vi "Hahn 2 Pulse Sequence Generator.vi"(4 "MW Delay":dbl, 5 "Optical Pulse Sequence":T1(array[cluster]), 6 "Tau' step size 2":dbl, 7 "No. Instructions":i32, 8 "Tau' max 2":dbl, 9 "Tau' min 2":dbl, 10 "Tau":dbl, 11 "Rabi Frequency  2":dbl) -> (2 "Tau'":dbl[](array[numeric]), 3 "Pulse Sequence":T1(array[cluster]))   [LabVIEW 2012]
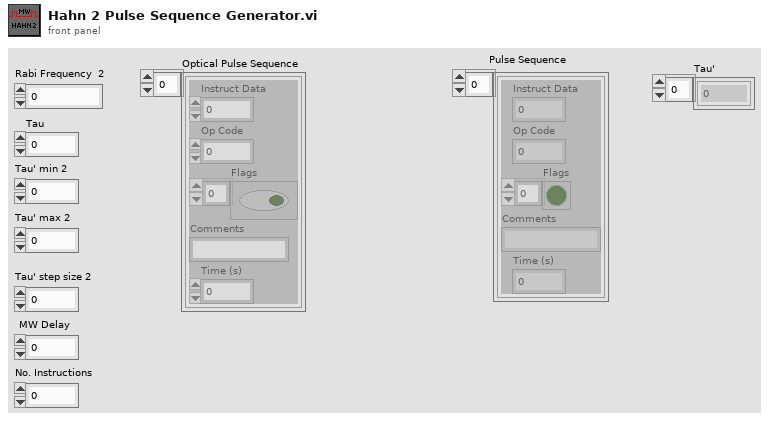
[diagram p1: front panel]
types:
  T1 = cluster{"Instruct Data":i32, "Op Code":i32, "Flags":bool[], "Comments":string, "Time (s)":dbl}[]
  T2 = cluster{"Instruct Data":i32, "Op Code":i32, "Flags":bool[], "Comments":string, "Time (s)":dbl}
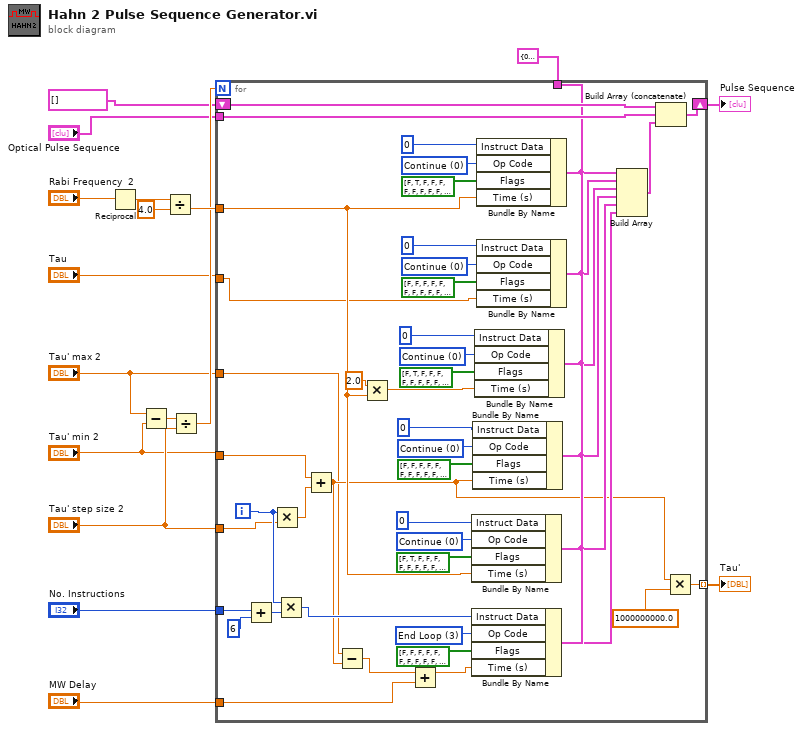
[diagram p0: block diagram]
diagram:
  n1 = Reciprocal(x="Rabi Frequency  2") -> (1/x=w16:dbl)
  n2 = Subtract(x="Tau' max 2", y="Tau' min 2") -> (x-y=w17:dbl)
  n3 = Divide(x=w16, y=4.0) -> (x/y=w15:dbl)
  n4 = Divide(x=w17, y="Tau' step size 2") -> (x/y=w12:dbl)
  n5 = for {
    N: w12 -> [_]
    tunnel: w15 -> [w43]
    shift-right: [w61] -> w2
    shift-left: T1 [] -> [w60]
    tunnel: "Optical Pulse Sequence" -> [w59]
    tunnel: T2 {"Instruct Data"=0, "Op Code"=0, "Flags"=[FALSE, FALSE, FALSE, FALSE, FALSE, FALSE, FALSE, FALSE, FALSE, FALSE, FALSE, FALSE, FALSE, FALSE, FALSE, FALSE, FALSE, FALSE, FALSE, FALSE, FALSE, TRUE, TRUE, TRUE], "Comments"="", "Time (s)"=0.01} ("PB Inst 2") -> [w40]
    tunnel: [w25] -> w1 mode=indexing
    tunnel: "Tau" -> [w24]
    tunnel: "Tau' step size 2" -> [w23]
    tunnel: "Tau' min 2" -> [w22]
    tunnel: "MW Delay" -> [w21]
    tunnel: "Tau' max 2" -> [w19]
    tunnel: "No. Instructions" -> [w18]
    i -> [w36]
    w41 = 3 items=["Continue", "Stop", "Loop", "End Loop", "JSR", "RTS", "Branch", "Long Delay", "Wait"] ("Op Code")
    w45 = 0 items=["Continue", "Stop", "Loop", "End Loop", "JSR", "RTS", "Branch", "Long Delay", "Wait"] ("Op Code")
    w48 = 0 items=["Continue", "Stop", "Loop", "End Loop", "JSR", "RTS", "Branch", "Long Delay", "Wait"] ("Op Code")
    w53 = 0 items=["Continue", "Stop", "Loop", "End Loop", "JSR", "RTS", "Branch", "Long Delay", "Wait"] ("Op Code")
    w57 = 0 items=["Continue", "Stop", "Loop", "End Loop", "JSR", "RTS", "Branch", "Long Delay", "Wait"] ("Op Code")
    w63 = 0 items=["Continue", "Stop", "Loop", "End Loop", "JSR", "RTS", "Branch", "Long Delay", "Wait"] ("Op Code")
    n6 = Add(x=w18, y=6) -> (x+y=w37:i32)
    n7 = Multiply(x=w36, y=w23) -> (x*y=w55:dbl)
    n8 = Multiply(x=w36, y=w37) -> (x*y=w35:i32)
    n9 = Add(x=w22, y=w55) -> (x+y=w26:dbl)
    n10 = Subtract(x=w19, y=w26) -> (x-y=w20:dbl)
    n11 = Multiply(x=2.0, y=w43) -> (x*y=w51:dbl)
    n12 = Add(x=w20, y=w21) -> (x+y=w39:dbl)
    n13 = Bundle By Name(cluster=w40, "Instruct Data"=0, "Op Code"=w45, "Flags"=bool[] [FALSE, TRUE, FALSE, FALSE, FALSE, FALSE, FALSE, FALSE, FALSE, FALSE, FALSE, FALSE, FALSE, FALSE, FALSE, FALSE, FALSE, FALSE, FALSE, FALSE, FALSE, TRUE, TRUE, TRUE], "Time (s)"=w43) -> (w31:T2)
    n14 = Bundle By Name(cluster=w40, "Instruct Data"=w35, "Op Code"=w41, "Flags"=bool[] [FALSE, FALSE, FALSE, FALSE, FALSE, FALSE, FALSE, FALSE, FALSE, FALSE, FALSE, FALSE, FALSE, FALSE, FALSE, FALSE, FALSE, FALSE, FALSE, FALSE, FALSE, TRUE, TRUE, TRUE], "Time (s)"=w39) -> (w32:T2)
    n15 = Bundle By Name(cluster=w40, "Instruct Data"=0, "Op Code"=w48, "Flags"=bool[] [FALSE, FALSE, FALSE, FALSE, FALSE, FALSE, FALSE, FALSE, FALSE, FALSE, FALSE, FALSE, FALSE, FALSE, FALSE, FALSE, FALSE, FALSE, FALSE, FALSE, FALSE, TRUE, TRUE, TRUE], "Time (s)"=w26) -> (w30:T2)
    n16 = Bundle By Name(cluster=w40, "Instruct Data"=0, "Op Code"=w53, "Flags"=bool[] [FALSE, TRUE, FALSE, FALSE, FALSE, FALSE, FALSE, FALSE, FALSE, FALSE, FALSE, FALSE, FALSE, FALSE, FALSE, FALSE, FALSE, FALSE, FALSE, FALSE, FALSE, TRUE, TRUE, TRUE], "Time (s)"=w51) -> (w29:T2)
    n17 = Bundle By Name(cluster=w40, "Instruct Data"=0, "Op Code"=w63, "Flags"=bool[] [FALSE, TRUE, FALSE, FALSE, FALSE, FALSE, FALSE, FALSE, FALSE, FALSE, FALSE, FALSE, FALSE, FALSE, FALSE, FALSE, FALSE, FALSE, FALSE, FALSE, FALSE, TRUE, TRUE, TRUE], "Time (s)"=w43) -> (w33:T2)
    n18 = Bundle By Name(cluster=w40, "Instruct Data"=0, "Op Code"=w57, "Flags"=bool[] [FALSE, FALSE, FALSE, FALSE, FALSE, FALSE, FALSE, FALSE, FALSE, FALSE, FALSE, FALSE, FALSE, FALSE, FALSE, FALSE, FALSE, FALSE, FALSE, FALSE, FALSE, TRUE, TRUE, TRUE], "Time (s)"=w24) -> (w28:T2)
    n19 = Build Array(w33, w28, w29, w30, w31, w32) -> (w34:T1)
    n20 = Build Array (concatenate)(w60, w59, w34) -> (w61:T1)
    n21 = Multiply(x=w26, y=1000000000.0) -> (x*y=w25:dbl)
  }
  "Pulse Sequence" <- w2
  "Tau'" <- w1
